vi "Configure Parameter DC.vi"() -> ()   [LabVIEW 2018, in "Fluke 9500B.lvlib"]
uses:
  <instrlib>/Fluke 9500B/Fluke 9500B.lvlib
panel:
  in  "STAT":enum16{"ON", "OFF"}(ring)
  in  "PARAM":enum16{"GRO", "MCH"}(ring)
  out "VISA resource name out":refnum<visa-resource-name>
  out "error out":errorcluster
  in  "error in (no error)":errorcluster
  in  "VISA resource name":refnum<visa-resource-name>
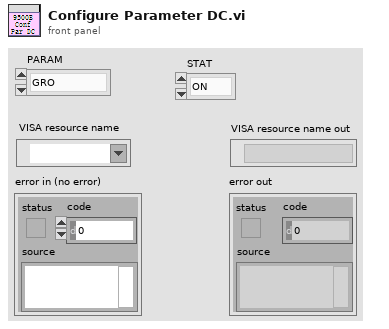
[diagram p1: front panel]
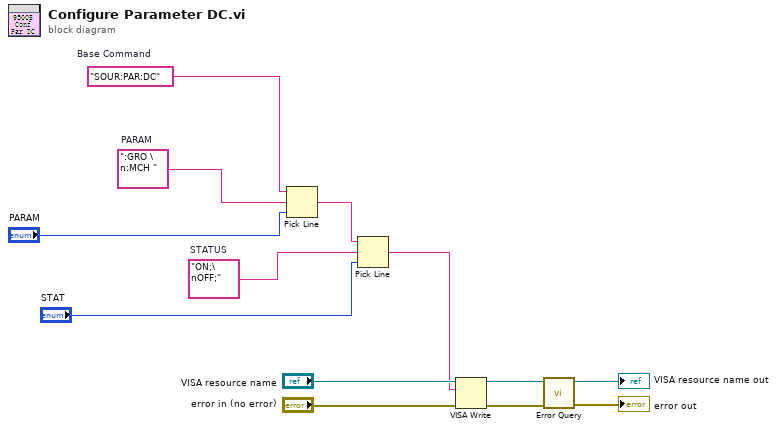
[diagram p0: block diagram]
diagram:
  w6 = "ON;\nOFF;"  # STATUS
  w10 = ":GRO \n:MCH "  # PARAM
  w11 = "SOUR:PAR:DC"  # Base Command
  n1 = Pick Line(string ("")=w11, multi-line string=w10, line index="PARAM") -> (output string=w8:string)
  n2 = Pick Line(string ("")=w8, multi-line string=w6, line index="STAT") -> (output string=w7:string)
  n3 = VISA Write(VISA resource name="VISA resource name", write buffer=w7, error in (no error)="error in (no error)") -> (VISA resource name out=w4:refnum<visa-resource-name>, error out=w3:errorcluster)  [unwired: 1 out]
  n4 = call <instrlib>:"Error Query.vi"("error in (no error)"=w3, "VISA resource name"=w4) -> ("error out"=→"error out":errorcluster, "VISA resource name out"=→"VISA resource name out":refnum<visa-resource-name>)  [unwired: 6 in, 2 out]
